vi "tm412_snapseries.vi"() -> ()   [LabVIEW 2011]
panel:
  out "Current Frame Timestamp":dbl
  out "Image":u16[][](graph)
  in  "Play":bool
  in  "Acquire":bool
  out "Current Frame Index":i32=-1
  in  "Frames to Capture":i32=100
  out "Camera Serial":string
  out "Camera Model":string
  out "Camera Version":string
  out "Total Frames":i32
  out "error out":errorcluster {"code" format="%.0x"}
  in  "quit":bool
  # "This is an example of how to capture\ndata at full speed to RAM, then read \nthe data from the buffer later."
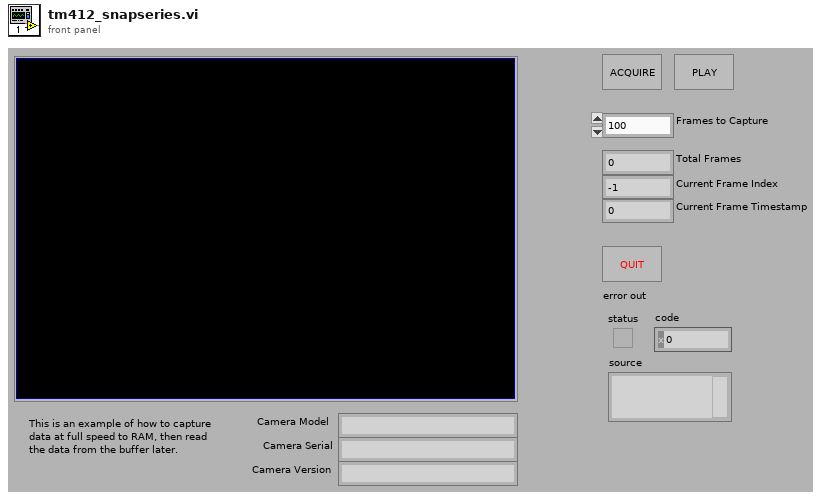
[diagram p1: front panel]
types:
  T1 = cluster{"Model":string, "Camera ID":string, "Firmware":string}
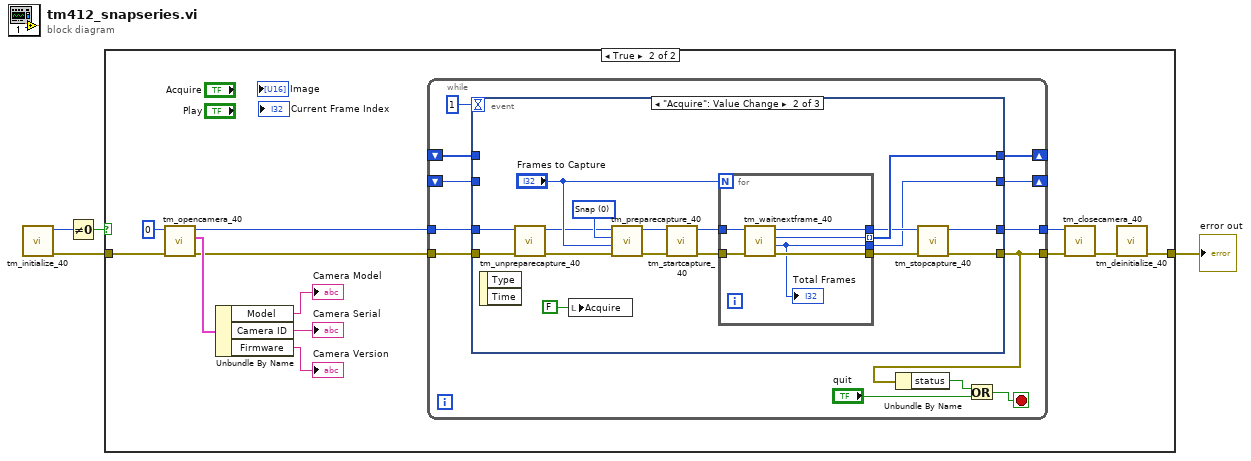
[diagram p0: block diagram]
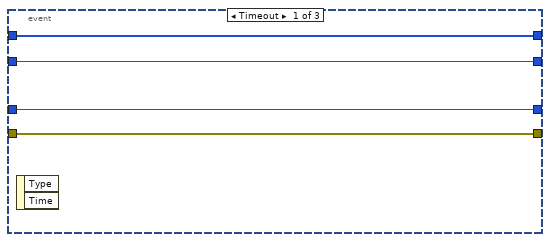
[diagram p3: hidden frame]
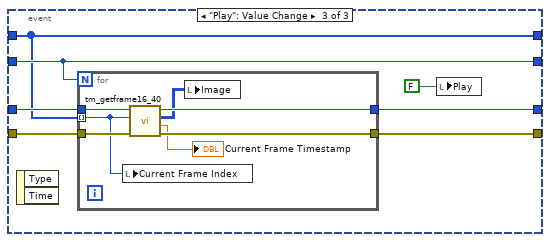
[diagram p4: hidden frame]
diagram:
  n1 = call <userlib>:"tm_initialize_40.vi"() -> ("error out"=w1:errorcluster, "Number Of Cameras"=w2:u32)  [unwired: 8 in, 2 out]
  n2 = Not Equal To 0?(x=w2) -> (x != 0?=w4:bool)
  n3 = case shown="True" w4 {
    tunnel: [w5 w14] -> w3
    tunnel: w1 -> [w5 w17]
    frame False {
    }
    frame True {
      n4 = call <userlib>:"tm_opencamera_40.vi"("error in (no error)"=w17, "Camera Index"=u32 0) -> ("error out"=w9:errorcluster, "Camera Details"=w10:T1, "Handle out"=w13:u32)  [unwired: 7 in]
      n5 = Unbundle By Name(w10) -> ("Model"=→"Camera Model":string, "Camera ID"=→"Camera Serial":string, "Firmware"=→"Camera Version":string)
      n6 = while {
        tunnel: [w22] -> w12
        tunnel: [w29] -> w11
        tunnel: w13 -> [w27]
        tunnel: w9 -> [w26]
        shift-right: [w18] -> _
        shift-left: _ -> [w25]
        shift-right: [w24] -> _
        shift-left: _ -> [w23]
        stop <- w19 stop-if-true
        n7 = event shown="[1] \"Acquire\": Value Change" {
          selector: _ -> [_ _ _]
          dyn-events: _ -> [_ _ _]
          timeout: 1 -> [_ _ _]
          tunnel: [w32 w41 w63] -> w29
          tunnel: [w33 w42 w62] -> w22
          tunnel: w26 -> [w33 w37 w60]
          tunnel: w27 -> [w32 w34 w61]
          tunnel: [w30 w38 w59] -> w18
          tunnel: w25 -> [w30 _ w59]
          tunnel: [w31 w45 w57] -> w24
          tunnel: w23 -> [w31 _ w57]
          event Timeout {
            n8 = event-data() -> ()  [unwired: 1 in, 2 out]
          }
          event "Acquire": Value Change {
            w46 = 0 items=["Snap", "Sequence"] ("Capture mode")
            n9 = event-data() -> ()  [unwired: 1 in, 2 out]
            n10 = call <userlib>:"tm_unpreparecapture_40.vi"("error in (no error)"=w37, "Handle in"=w34) -> ("error out"=w36:errorcluster, "Handle out"=w35:u32)  [unwired: 8 in]
            n11 = local write "Acquire"(FALSE) -> ()
            n12 = call <userlib>:"tm_preparecapture_40.vi"("error in (no error)"=w36, "Frames"="Frames to Capture", "Capture mode"=w46, "Handle in"=w35) -> ("error out"=w47:errorcluster, "Handle out"=w48:u32)  [unwired: 4 in, 2 out]
            n13 = call <userlib>:"tm_startcapture_40.vi"("error in (no error)"=w47, "Handle in"=w48) -> ("error out"=w49:errorcluster, "Handle out"=w50:u32)  [unwired: 8 in]
            n14 = for {
              N: "Frames to Capture" -> [_]
              tunnel: w49 -> [w55]
              tunnel: w50 -> [w56]
              tunnel: [w53] -> w45 mode=indexing
              tunnel: [w54] -> w40
              tunnel: [w51] -> w38
              tunnel: [w52] -> w39
              n15 = call <userlib>:"tm_waitnextframe_40.vi"("error in (no error)"=w55, "Handle in"=w56) -> ("error out"=w52:errorcluster, "Frame Count"=w51:i32, "Frame Index"=w53:i32, "Handle out"=w54:u32)  [unwired: 6 in]
              "Total Frames" <- w51
            }
            n16 = call <userlib>:"tm_stopcapture_40.vi"("error in (no error)"=w39, "Handle in"=w40) -> ("error out"=w42:errorcluster, "Handle out"=w41:u32)  [unwired: 8 in]
          }
          event "Play": Value Change {
            n17 = event-data() -> ()  [unwired: 1 in, 2 out]
            n18 = for {
              N: w59 -> [_]
              tunnel: w57 -> [w65] mode=indexing
              tunnel: w60 -> [w70]
              tunnel: w61 -> [w69]
              tunnel: [w68] -> w62
              tunnel: [w67] -> w63
              n19 = local write "Current Frame Index"(w65) -> ()
              n20 = call <userlib>:"tm_getframe16_40.vi"("error in (no error)"=w70, "Frame Index"=w65, "Handle in"=w69) -> ("error out"=w68:errorcluster, "Timestamp"=→"Current Frame Timestamp":dbl, "Data"=w66:u16[][], "Handle out"=w67:u32)  [unwired: 5 in]
              n21 = local write "Image"(w66) -> ()
            }
            n22 = local write "Play"(FALSE) -> ()
          }
        }
        n23 = Unbundle By Name(w22) -> ("status"=w21:bool)
        n24 = Or(x=w21, y="quit") -> (x .or. y?=w19:bool)
      }
      n25 = call <userlib>:"tm_closecamera_40.vi"("error in (no error)"=w12, "Handle in"=w11) -> ("error out"=w15:errorcluster)  [unwired: 9 in]
      n26 = call <userlib>:"tm_deinitialize_40.vi"("error in (no error)"=w15) -> ("error out"=w14:errorcluster)  [unwired: 10 in]
    }
  }
  "error out" <- w3
